vi "Stop.vi"(8 "error in":errorcluster, 11 "Control Load CFG in":refnum<class "EL Control Load CFG.lvclass">) -> (0 "error out":errorcluster, 3 "Control Load CFG out":refnum<class "EL Control Load CFG.lvclass">)   [LabVIEW 2023, in "EL Control Load CFG.lvclass"]
uses:
  EL Control Load CFG.lvclass
  SCPI PE Input.ctl
  EL Control Load CFG.lvclass/EL Control Load CFG.ctl
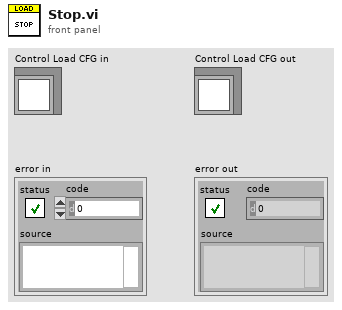
[diagram p1: front panel]
types:
  T1 = typedef "SCPI PE Input.ctl" = cluster{"Action":enum16{"Write", "Query"}, "SCPI":string}
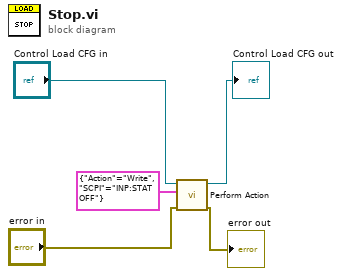
[diagram p0: block diagram]
diagram:
  n1 = call-dynamic "Perform Action.vi"("error in"="error in", "Input"=T1 {"Action"=enum."Write", "SCPI"="INP:STAT OFF"} ("PE Input"), "Control Load CFG in"="Control Load CFG in") -> ("error out"=→"error out":errorcluster, "Control Load CFG out"=→"Control Load CFG out":refnum<class "EL Control Load CFG.lvclass">)  [unwired: 6 in, 1 out]
